vi "is_done.vi"(8 "error in (no error)":errorcluster, 11 "Analog_Input (in)":refnum<class "Analog_Input.lvclass">) -> (0 "error out":errorcluster, 2 "task done?":bool, 3 "Analog_Input":refnum<class "Analog_Input.lvclass">)   [LabVIEW 2013, in "Analog_Input.lvclass"]
uses:
  Analog_Input.lvclass
  Analog_Input.lvclass/Analog_Input.ctl
  Globals.vi
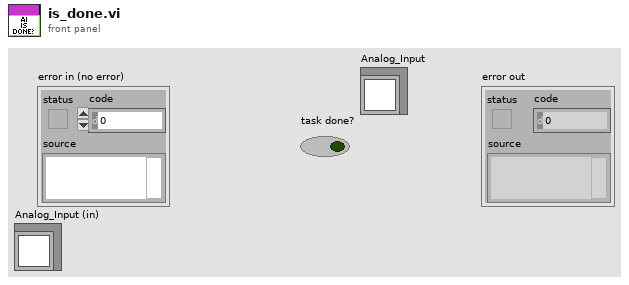
[diagram p1: front panel]
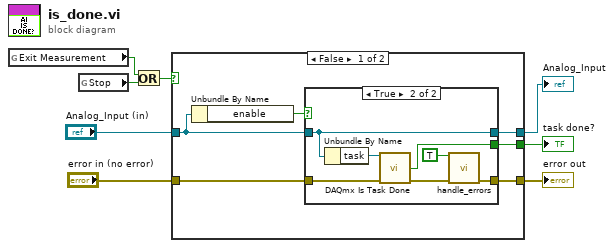
[diagram p0: block diagram]
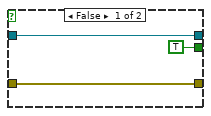
[diagram p2: hidden frame]
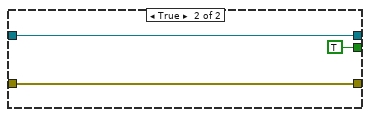
[diagram p3: hidden frame]
diagram:
  n1 = global read "Globals.vi" "Exit Measurement"() -> (w7:bool)
  n2 = global read "Globals.vi" "Stop"() -> (w6:bool)
  n3 = Or(x=w7, y=w6) -> (x .or. y?=w5:bool)
  n4 = case shown="False" w5 {
    tunnel: [w13 w26] -> w8
    tunnel: [w9 w27] -> w1
    tunnel: "Analog_Input (in)" -> [w10 w27]
    tunnel: "error in (no error)" -> [w12 w26]
    tunnel: [w11 TRUE ("Exit Measurement")] -> w3
    frame False {
      n5 = Unbundle By Name(w10) -> ("enable"=w14:bool)
      n6 = case shown="True" w14 {
        tunnel: w12 -> [w17 w24]
        tunnel: [w17 w21] -> w13
        tunnel: [TRUE ("task done?") w23] -> w11
        tunnel: w10 -> [w15 w18]
        tunnel: [w15 w18] -> w9
        frame False {
        }
        frame True {
          n7 = Unbundle By Name(w18) -> ("task"=w19:refnum<k21>)
          n8 = call <vilib>:"DAQmx Is Task Done.vi"("task/channels in"=w19, "error in"=w24) -> ("task done?"=w23:bool, "error out"=w22:errorcluster)  [unwired: 11 in, 1 out]
          n9 = call "handle_errors.vi"("Exit Operation"=TRUE ("Exit Measurement"), "error in (no error)"=w22) -> ("error out"=w21:errorcluster)  [unwired: 13 in]
        }
      }
    }
    frame True {
    }
  }
  "error out" <- w8
  "task done?" <- w3
  "Analog_Input" <- w1
